vi "rs3 get stream intrinsics3.vi"(8 "error in (no error)":errorcluster, 11 "stream profile":u64) -> (0 "error out":errorcluster, 1 "intrin out":T1 {"model" items=["RS_DISTORTION_NONE", "RS_DISTORTION_MODIFIED_BROWN_CONRADY", "RS_DISTORTION_INVERSE_BROWN_CONRADY", "RS_DISTORTION_FTHETA", "RS_DISTORTION_BROWN_CONRADY", "RS_DISTORTION_COUNT"]}, 2 "error":u64, 3 "stream profile out":u64)   [LabVIEW 2017, in "libRealSense3.lvlib"]
doc: "Returns the sensor streams intrinsics\n int width; /* width of the image in pixels */\n int height; /* height of the image in pixels */\n float ppx; /* horizontal coordinate of the principal point of the image, as a pixel offset from the left edge */\n float ppy; /* vertical coordinate of the principal point of the image, as a pixel offset from the top edge */\n float fx; /* focal length of the image plane, as a multiple of pixel width */\n float fy; /* focal length of the image plane, as a multiple of pixel height */\n rs_distortion model; /* distortion model of the image */\n float coeffs[5]; /* distortion coefficients */\n\n\nNote that the intrinsic focal points and principle points are in units of pixels. This will change for different resolutions. \nThe distortion model is how the lens was modelled."
uses:
  libRealSense3.lvlib
panel:
  # "RS3 Get Stream Intrinsics3"
  # "(C) Intel Corp. 2017,  AGJ"
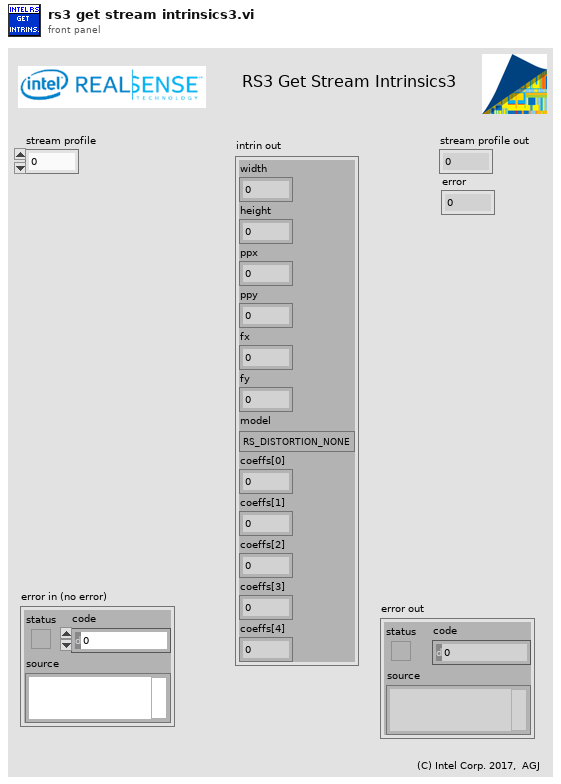
[diagram p1: front panel]
types:
  T1 = cluster{"width":i32, "height":i32, "ppx":sgl, "ppy":sgl, "fx":sgl, "fy":sgl, "model":u32, "coeffs[0]":sgl, "coeffs[1]":sgl, "coeffs[2]":sgl, "coeffs[3]":sgl, "coeffs[4]":sgl}
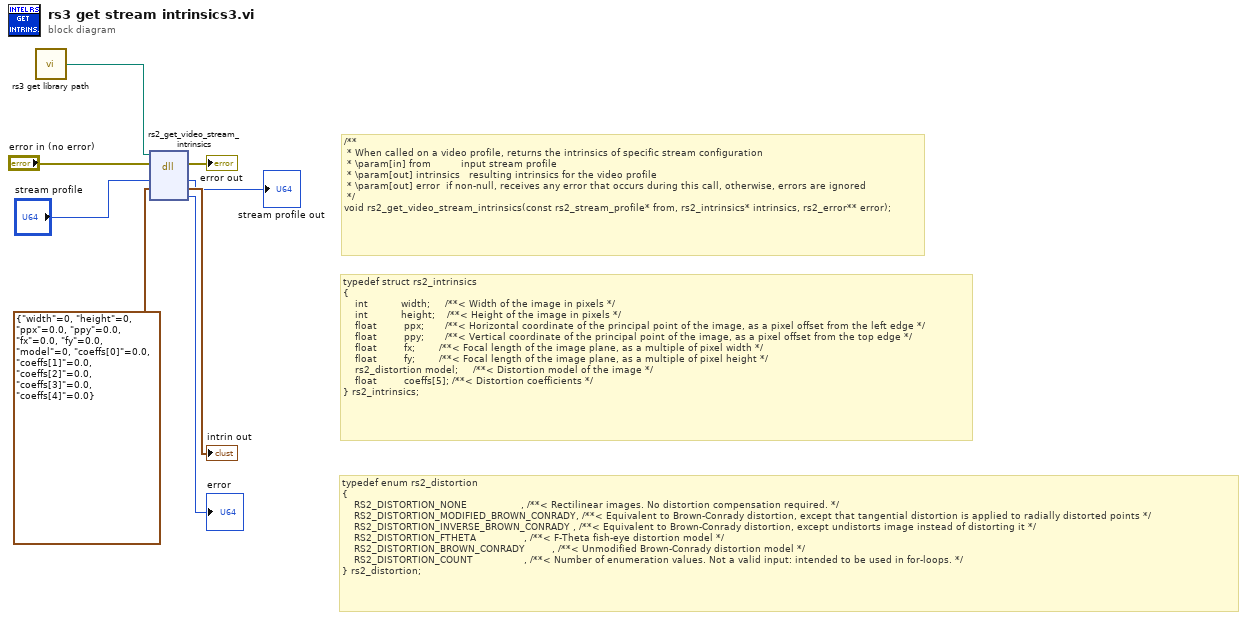
[diagram p0: block diagram]
diagram:
  # "typedef enum rs2_distortion\n{\n    RS2_DISTORTION_NONE                  , /**< Rectilinear images. No distortion compensation required. */\n    RS2_DISTORTION_MODIFIED_BROWN_CONRADY, /**< Equivalent to Brown-Conrady distortion, except that tangential distortion is applied to radially distorted points */\n    RS2_DISTORTION_INVERSE_BROWN_CONRADY , /**< Equivalent to Brown-Conrady distortion, except undistorts image instead of distorting it */\n    RS2_DISTORTION_FTHETA                , /**< F-Theta fish-eye distortion model */\n    RS2_DISTORTION_BROWN_CONRADY         , /**< Unmodified Brown-Conrady distortion model */\n    RS2_DISTORTION_COUNT                 , /**< Number of enumeration values. Not a valid input: intended to be used in for-loops. */\n} rs2_distortion;"
  # "typedef struct rs2_intrinsics\n{\n    int           width;     /**< Width of the image in pixels */\n    int           height;    /**< Height of the image in pixels */\n    float         ppx;       /**< Horizontal coordinate of the principal point of the image, as a pixel offset from the left edge */\n    float         ppy;       /**< Vertical coordinate of the principal point of the image, as a pixel offset from the top edge */\n    float         fx;        /**< Focal length of the image plane, as a multiple of pixel width */\n    float         fy;        /**< Focal length of the image plane, as a multiple of pixel height */\n    rs2_distortion model;     /**< Distortion model of the image */\n    float         coeffs[5]; /**< Distortion coefficients */\n} rs2_intrinsics;"
  # "/**\n * When called on a video profile, returns the intrinsics of specific stream configuration\n * \\param[in] from          input stream profile\n * \\param[out] intrinsics   resulting intrinsics for the video profile\n * \\param[out] error  if non-null, receives any error that occurs during this call, otherwise, errors are ignored\n */\nvoid rs2_get_video_stream_intrinsics(const rs2_stream_profile* from, rs2_intrinsics* intrinsics, rs2_error** error);"
  n1 = call "rs3 get library path.vi"() -> ("Realsense 2 Library Path"=w1:path)
  n2 = dll-call lib="C:/Users/agrunnet/Documents/libRealSense6/realsense2.dll" fn="rs2_get_video_stream_intrinsics"(path in=w1, error in="error in (no error)", "stream profile"="stream profile", "intrinsics"=T1 {"width"=0, "height"=0, "ppx"=0.0, "ppy"=0.0, "fx"=0.0, "fy"=0.0, "model"=0, "coeffs[0]"=0.0, "coeffs[1]"=0.0, "coeffs[2]"=0.0, "coeffs[3]"=0.0, "coeffs[4]"=0.0} ("intrin")) -> (error out=→"error out":errorcluster, "stream profile"=→"stream profile out":u64, "intrinsics"=→"intrin out":T1, "error"=→"error":u64)  [unwired: 3 in, 1 out]
